vi "DB Tools Database Transaction.vi"   [LabVIEW 2017, in "NI_Database_API.lvlib"]
doc: "Begins, commits, or rolls back a transaction for any type of reference. Wire data to the reference input to determine the polymorphic instance to use or manually select the instance."
uses:
  <vilib>/addons/database/NI_Database_API.lvlib
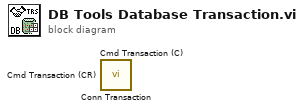
[diagram p0: block diagram]
diagram:
  n1 = call <vilib>:"Conn Transaction.vi"() -> ()  [unwired: 6 in, 2 out]
  n2 = call <vilib>:"Cmd Transaction (C).vi"() -> ()  [unwired: 6 in, 2 out]
  n3 = call <vilib>:"Cmd Transaction (CR).vi"() -> ()  [unwired: 6 in, 2 out]
